vi "IV-Trace_v1.0.vi"() -> ()   [LabVIEW 2014]
doc: "This example shows how to configure a measurement and take a reading."
uses:
  <instrlib>/Keithley 24XX/Public/Data/Read (Single Point).vi
  <instrlib>/Keithley 24XX/Keithley 24XX.lvlib
panel:
  out "Data Resistivity":string
  in  "Data Resistivity":path=path "C:/Users/Administrator/Documents/Device-characterization-setup/IV-Trace/Data/dumb/2015_xx_xx_xxxx_xx_keithley_resistivity_001.txt"
  out "Resistance-Voltage":cluster{sgl[], sgl[]}(graph)
  in  "current multiplier":dbl=1.0
  out "Data IV Keithley":string
  in  "Data IV Keithley":path=path "C:/Users/Administrator/Documents/Device-characterization-setup/IV-Trace/Data/dumb/2015_xx_xx_xxxx_xx_keithley_001.txt"
  out "IV Curve":cluster{sgl[], dbl[]}(graph)
  in  "Stop Voltage/Current":dbl=2.0
  in  "Step":dbl=1.0
  in  "Source Mode  (0: Voltage)":u16(ring) items=["Voltage", "Current"]
  in  "Compliance  Level (0.1)":dbl=1.0
  in  "Start Voltage/Current":dbl
  in  "Enable Resistance Auto Range (T:Enable)":bool
  in  "Enable Current Auto Range (T:Enable)":bool=TRUE
  in  "Enable Voltage Auto Range (T:Enable)":bool
  in  "Resistance Manual Range (1.0)":dbl=1.0
  in  "Current Manual Range (1.0)":dbl=1.0
  in  "Voltage Manual Range (1.0)":dbl=1.0
  out "Resistance":sgl
  out "Current":sgl
  out "Voltage":sgl
  in  "Serial Configuration":T1={"Baud Rate"=9600, "Parity"=0, "Data Bits"=8, "Stop Bits"=10, "Flow Control"=0} {"Flow Control" items=["None", "XON/XOFF", "RTS/CTS", "XON/XOFF & RTS/CTS", "DTR/DSR", "XON/XOFF & DTR/DSR"]; "Stop Bits" items=["1.0"=10, "1.5"=15, "2.0"=20]; "Data Bits" items=["7"=7, "8"=8]; "Parity" items=["None", "Odd", "Even", "Mark", "Space"]; "Baud Rate" items=["300"=300, "600"=600, "1200"=1200, "2400"=2400, "4800"=4800, "9600"=9600, "19200"=19200]}
  in  "VISA resource name":refnum<visa-resource-name>="GPIB9::24::INSTR"
  # "NanoBEEs 2015-IV Tracer v1.0"
  # "Source Settings"
  # "GPIB9::24::INSTR"
  # "Voltage Range Settings"
  # "Current Range Settings"
  # "This multiplies the current value\nwith the number that entered, in order\nto  graph lower current values."
  # "Resistance Range Settings"
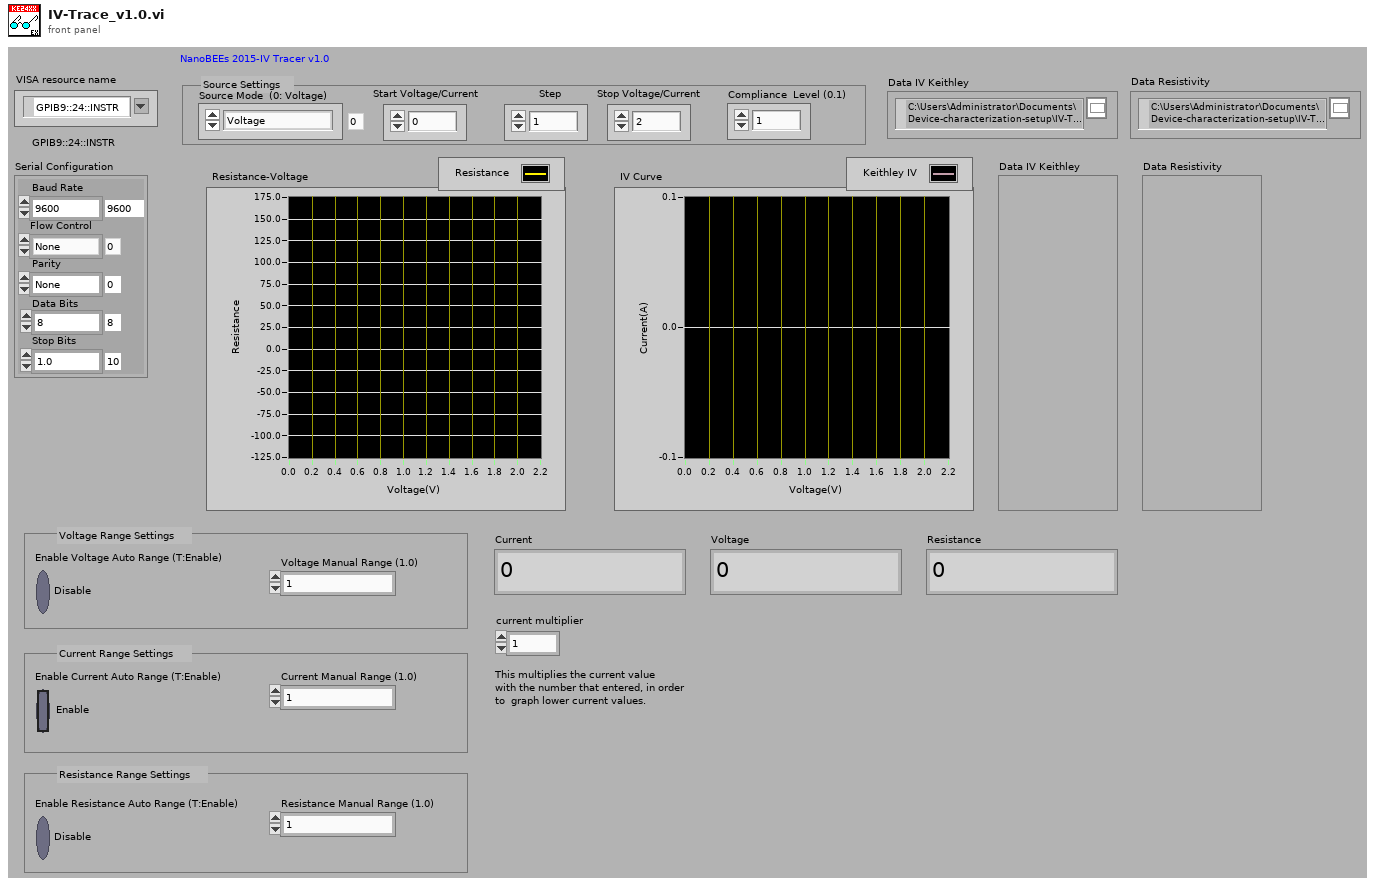
[diagram p1: front panel]
types:
  T1 = cluster{"Baud Rate":u32, "Parity":u16, "Data Bits":u16, "Stop Bits":u16, "Flow Control":u16}
  T2 = enum16{"open", "replace", "create", "open or create", "replace or create", "replace or create with confirmation"}
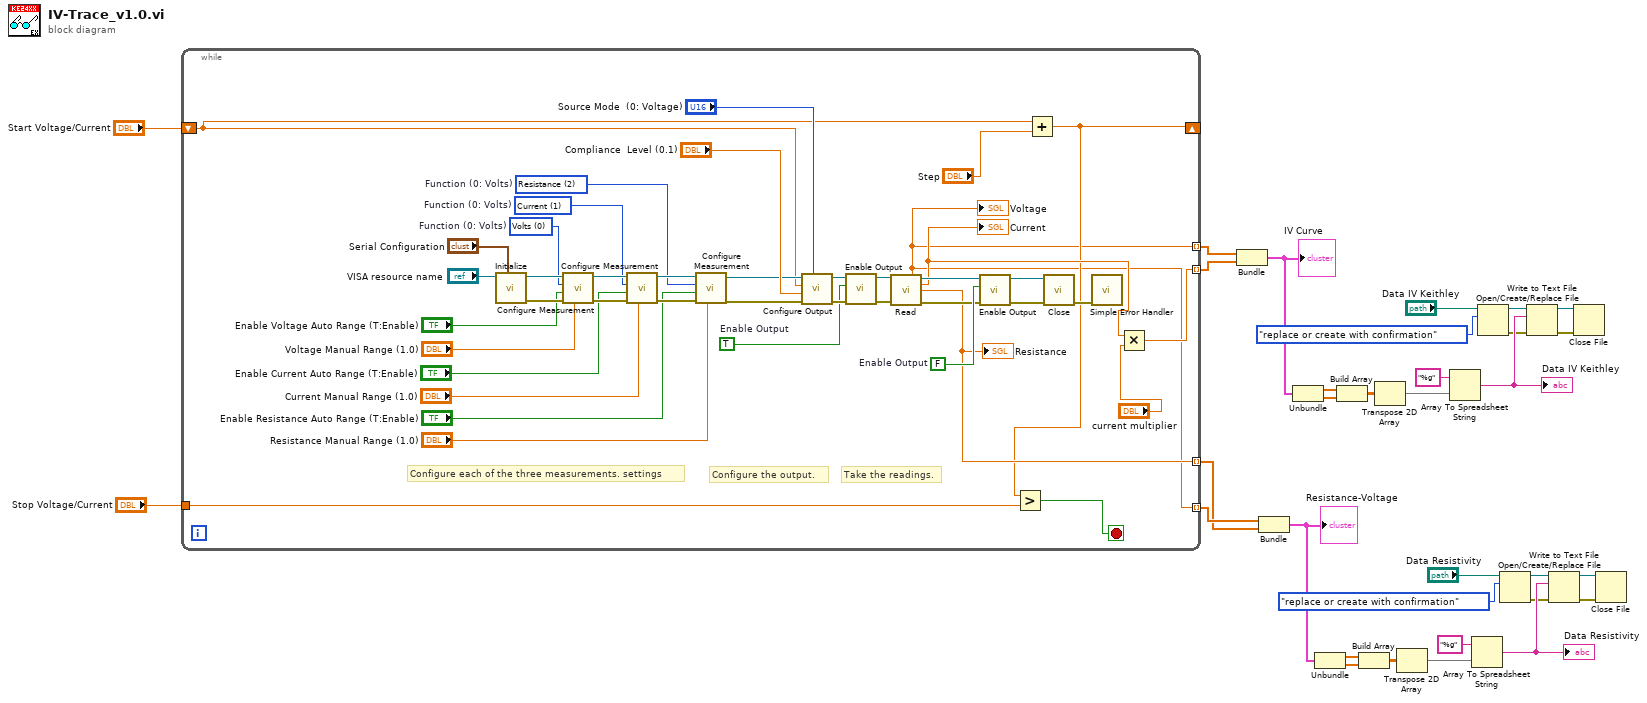
[diagram p0: block diagram]
diagram:
  n1 = while {
    shift-right: [w34] -> _
    shift-left: "Start Voltage/Current" -> [w41]
    tunnel: "Stop Voltage/Current" -> [w39]
    tunnel: [w36] -> w17 mode=indexing
    tunnel: [w33] -> w16 mode=indexing
    tunnel: [w38] -> w1 mode=indexing
    tunnel: [w33] -> w2 mode=indexing
    stop <- w42 stop-if-true
    w46 = TRUE  # Enable Output
    w56 = FALSE  # Enable Output
    w63 = u16 2 items=["Volts", "Current", "Resistance"]  # Function (0: Volts)
    w64 = u16 1 items=["Volts", "Current", "Resistance"]  # Function (0: Volts)
    w65 = u16 0 items=["Volts", "Current", "Resistance"]  # Function (0: Volts)
    # "Take the readings."
    # "Configure the output."
    # "Configure each of the three measurements. settings"
    n2 = call <instrlib>:"Initialize.vi"("Serial Configuration"="Serial Configuration", "VISA resource name"="VISA resource name") -> ("error out"=w70:errorcluster, "VISA resource name out"=w71:refnum<visa-resource-name>)  [unwired: 8 in]
    n3 = call <instrlib>:"Configure Measurement.vi"("Manual Range (1.0)"="Voltage Manual Range (1.0)", "error in (no error)"=w70, "Enable Auto Range (T:Enable)"="Enable Voltage Auto Range (T:Enable)", "Function (0: Volts)"=w65, "VISA resource name"=w71) -> ("error out"=w68:errorcluster, "VISA resource name out"=w69:refnum<visa-resource-name>)  [unwired: 5 in]
    n4 = call <instrlib>:"Configure Measurement.vi"("Manual Range (1.0)"="Current Manual Range (1.0)", "error in (no error)"=w68, "Enable Auto Range (T:Enable)"="Enable Current Auto Range (T:Enable)", "Function (0: Volts)"=w64, "VISA resource name"=w69) -> ("error out"=w67:errorcluster, "VISA resource name out"=w66:refnum<visa-resource-name>)  [unwired: 5 in]
    n5 = call <instrlib>:"Configure Measurement.vi"("Manual Range (1.0)"="Resistance Manual Range (1.0)", "error in (no error)"=w67, "Enable Auto Range (T:Enable)"="Enable Resistance Auto Range (T:Enable)", "Function (0: Volts)"=w63, "VISA resource name"=w66) -> ("error out"=w45:errorcluster, "VISA resource name out"=w44:refnum<visa-resource-name>)  [unwired: 5 in]
    n6 = call <instrlib>:"Configure Output.vi"("Source Mode  (0: Voltage)"="Source Mode  (0: Voltage)", "error in (no error)"=w45, "Compliance  Level (0.1)"="Compliance  Level (0.1)", "Output Level (0)"=w41, "VISA resource name"=w44) -> ("error out"=w47:errorcluster, "VISA resource name out"=w48:refnum<visa-resource-name>)  [unwired: 5 in]
    n7 = call <instrlib>:"Enable Output.vi"("error in (no error)"=w47, "Enable Output (T: Enable)"=w46, "VISA resource name"=w48) -> ("error out"=w50:errorcluster, "VISA resource name out"=w49:refnum<visa-resource-name>)  [unwired: 7 in]
    n8 = call-poly <instrlib>:"Read.vi"("VISA resource name"=w49, "error in (no error)"=w50) -> ("Voltage"=w33:sgl, "VISA resource name out"=w51:refnum<visa-resource-name>, "Current"=w37:sgl, "Resistance"=w38:sgl, "error out"=w52:errorcluster)  [unwired: 7 in, 2 out]
    "Voltage" <- w33
    "Current" <- w37
    "Resistance" <- w38
    n9 = call <instrlib>:"Enable Output.vi"("error in (no error)"=w52, "Enable Output (T: Enable)"=w56, "VISA resource name"=w51) -> ("error out"=w53:errorcluster, "VISA resource name out"=w54:refnum<visa-resource-name>)  [unwired: 7 in]
    n10 = Add(x=w41, y="Step") -> (x+y=w34:dbl)
    n11 = Greater?(x=w34, y=w39) -> (0:w42:bool)
    n12 = call <instrlib>:"Close.vi"("error in (no error)"=w53, "VISA resource name"=w54) -> ("error out"=w74:errorcluster)  [unwired: 9 in]
    n13 = call <vilib>:"Simple Error Handler.vi"("error in (no error)"=w74) -> ()  [unwired: 4 in, 5 out]
    n14 = Multiply(x=w37, y="current multiplier") -> (x*y=w36:dbl)
  }
  n15 = Bundle(w16, w17) -> (w24:cluster{sgl[], dbl[]})  [unwired: 1 out]
  "IV Curve" <- w24
  n16 = Bundle(w2, w1) -> (w9:cluster{sgl[], sgl[]})  [unwired: 1 out]
  "Resistance-Voltage" <- w9
  n17 = Unbundle(w24) -> (w25:sgl[], w26:dbl[])
  n18 = Unbundle(w9) -> (w10:sgl[], w11:sgl[])
  n19 = Build Array(w25, w26) -> (w27:dbl[][])
  n20 = Build Array(w10, w11) -> (w12:sgl[][])
  n21 = Transpose 2D Array(2D array=w27) -> (transposed array=w29:dbl[][])
  n22 = Transpose 2D Array(2D array=w12) -> (transposed array=w14:sgl[][])
  n23 = Array To Spreadsheet String(array=w29, 3:"%g" ("format string")) -> (spreadsheet string=w30:string)  [unwired: 1 in]
  "Data IV Keithley" <- w30
  n24 = Array To Spreadsheet String(array=w14, 3:"%g" ("format string")) -> (spreadsheet string=w15:string)  [unwired: 1 in]
  "Data Resistivity" <- w15
  n25 = Open/Create/Replace File(file path (use dialog)="Data IV Keithley", operation (0:open)=T2."replace or create with confirmation") -> (refnum out=w23:refnum<file>, error out=w18:errorcluster)  [unwired: 4 in, 1 out]
  n26 = Open/Create/Replace File(file path (use dialog)="Data Resistivity", operation (0:open)=T2."replace or create with confirmation") -> (refnum out=w8:refnum<file>, error out=w3:errorcluster)  [unwired: 4 in, 1 out]
  n27 = Write to Text File(file (use dialog)=w23, text=w30, error in=w18) -> (refnum out=w20:refnum<file>, error out=w19:errorcluster)  [unwired: 2 out]
  n28 = Write to Text File(file (use dialog)=w8, text=w15, error in=w3) -> (refnum out=w5:refnum<file>, error out=w4:errorcluster)  [unwired: 2 out]
  n29 = Close File(refnum=w20, error in=w19) -> ()  [unwired: 2 out]
  n30 = Close File(refnum=w5, error in=w4) -> ()  [unwired: 2 out]
